vi "Update Configuration with Existing Modules.vi"(7 "Module IDs":string[](array[string]), 8 "error in":errorcluster, 9 "default error responses":T1={"unknown"={"clear"=TRUE, "notify"=TRUE, "log"=FALSE, "remove module"=FALSE, "abort engine"=FALSE, "go to safe state"=FALSE, "recover module"=FALSE}, "trivial"={"clear"=TRUE, "notify"=TRUE, "log"=FALSE, "remove module"=FALSE, "abort engine"=FALSE, "go to safe state"=FALSE, "recover module"=FALSE}, "critical"={"clear"=TRUE, "notify"=TRUE, "log"=FALSE, "remove module"=FALSE, "abort engine"=FALSE, "go to safe state"=FALSE, "recover module"=FALSE}, "recoverable"={"clear"=TRUE, "notify"=TRUE, "log"=FALSE, "remove module"=FALSE, "abort engine"=FALSE, "go to safe state"=FALSE, "recover module"=FALSE}}, 10 "Default Module Decimation":T3={"Decimation"=1, "Offset"=0, "sort order"=0, "async?"=FALSE}, 11 "Standard Engine Configuration in":refnum<class "Standard Engine Configuration.lvclass">) -> (0 "error out":errorcluster, 3 "Standard Engine Configuration out":refnum<class "Standard Engine Configuration.lvclass">)   [LabVIEW 2013, in "Standard Engine Configuration.lvclass"]
doc: "This VI synchronizes its module specific configuration information with the list of modules specified by 'Module IDs'. \n\nIf more modules are specified in 'Module IDs' than exist already in the module-specific configuration, than a new element is created for each new Module ID based on the 'Default Module Decimation' and 'Default Module Error Configuration' inputs. \n\nIf the module specific configuration contains elements not present in the 'Module IDs' input, the additional configurations are deleted."
uses:
  Standard Engine Configuration.lvclass
  Module Decimation.ctl
  Runtime/error responses.ctl
  error options.ctl
  Standard Engine Configuration.lvclass/Standard Engine Configuration.ctl
  Find Module Specific Config.vi
  <vilib>/NI/Configuration Framework/error generator/NISE_error generator.vi
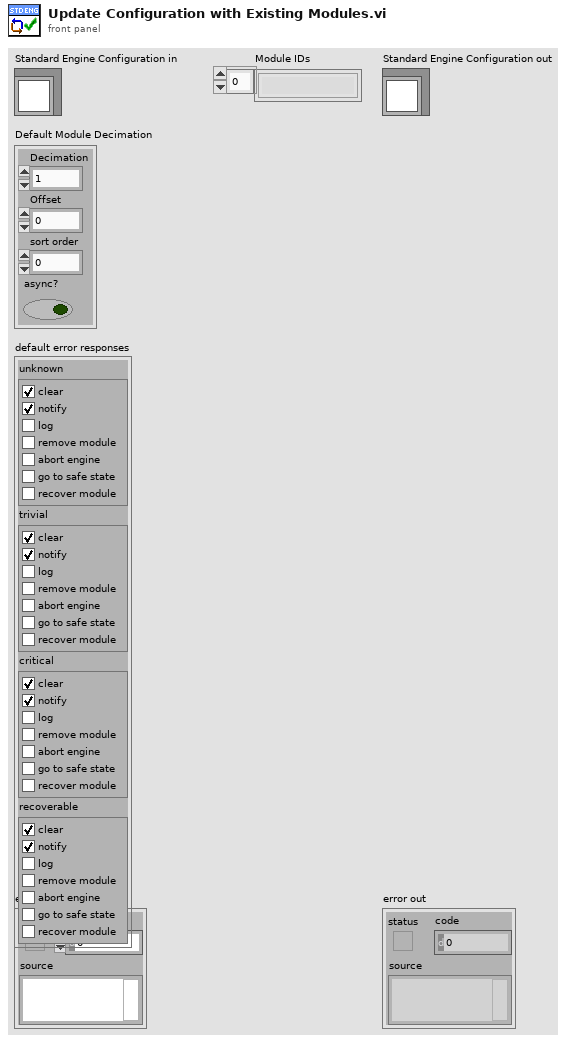
[diagram p1: front panel]
types:
  T1 = typedef "Standard Engine Configuration.lvclass/error responses.ctl" = cluster{"unknown":T2, "trivial":T2, "critical":T2, "recoverable":T2}
  T2 = typedef "Standard Engine Configuration.lvclass/error options.ctl" = cluster{"clear":bool, "notify":bool, "log":bool, "remove module":bool, "abort engine":bool, "go to safe state":bool, "recover module":bool}
  T3 = typedef "Standard Engine Configuration.lvclass/Module Decimation.ctl" = cluster{"Decimation":u16, "Offset":u16, "sort order":i32, "async?":bool}
  T4 = typedef "Standard Engine Configuration.lvclass/Module Specific Configuration.ctl" = cluster{"Module ID":string, "Module Decimation":T3, "error tag":string, "error responses":T1}
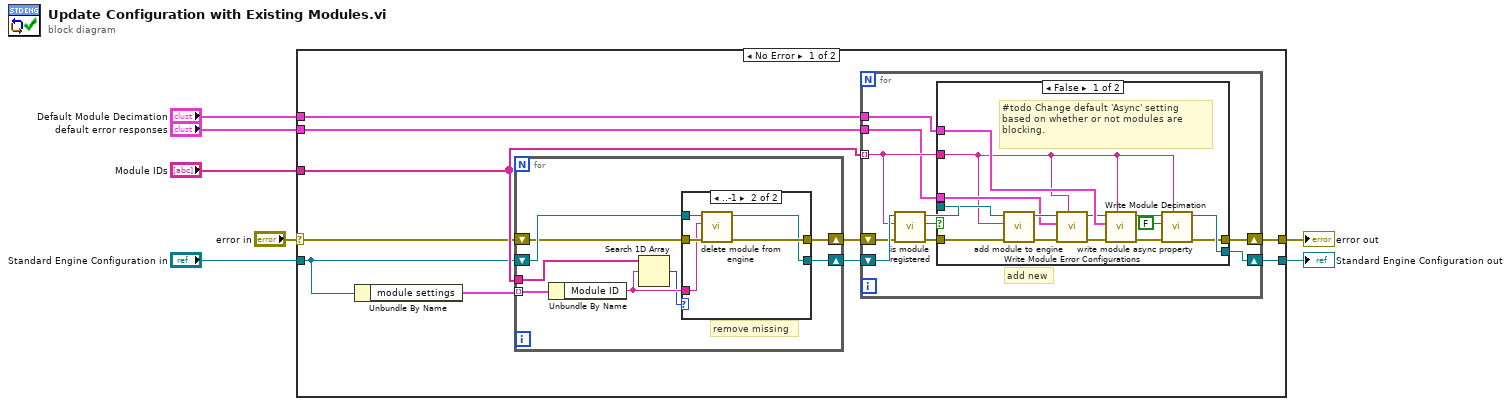
[diagram p0: block diagram]
diagram:
  n1 = case shown="No Error" "error in" {
    selector: "error in" -> [w11 w60]
    tunnel: [w15 w60] -> w6
    tunnel: [w16 w59] -> w4
    tunnel: "Standard Engine Configuration in" -> [w12 w59]
    tunnel: "Module IDs" -> [w13 _]
    tunnel: "Default Module Decimation" -> [w17 _]
    tunnel: "default error responses" -> [w8 _]
    frame No Error {
      n2 = Unbundle By Name(w12) -> ("module settings"=w14:T4[])
      n3 = for {
        tunnel: w14 -> [w25] mode=indexing
        tunnel: w13 -> [w24]
        shift-right: [w20] -> w10
        shift-left: w12 -> [w23]
        shift-right: [w21] -> w9
        shift-left: w11 -> [w22]
        # "remove missing"
        n4 = Unbundle By Name(w25) -> ("Module ID"=w19:string)
        n5 = Search 1D Array(1D array=w24, element=w19) -> (index of element=w18:i32)  [unwired: 1 in]
        n6 = case shown="..-1" w18 {
          tunnel: w23 -> [w27 w32]
          tunnel: w22 -> [w26 w31]
          tunnel: [w26 w30] -> w21
          tunnel: [w27 w29] -> w20
          tunnel: w19 -> [_ w28]
          frame 0.. {
          }
          frame ..-1 {
            n7 = call-dynamic "delete module from engine.vi"("error in"=w31, "module ID"=w28, "Standard Engine Configuration in"=w32) -> ("error out"=w30:errorcluster, "Standard Engine Configuration out"=w29:refnum<class "Standard Engine Configuration.lvclass">)  [unwired: 7 in]
          }
        }
      }
      n8 = for {
        shift-right: [w38] -> w15
        shift-left: w9 -> [w41]
        shift-right: [w39] -> w16
        shift-left: w10 -> [w42]
        tunnel: w13 -> [w36] mode=indexing
        tunnel: w17 -> [w34]
        tunnel: w8 -> [w33]
        # "add new"
        n9 = call-dynamic "is module registered.vi"("error in"=w41, "module ID"=w36, "engine configuration in"=w42) -> ("error out"=w37:errorcluster, "registered?"=w35:bool, "engine configuration out"=w40:refnum<class "Standard Engine Configuration.lvclass">)  [unwired: 6 in]
        n10 = case shown="False" w35 {
          tunnel: w40 -> [w56 w58]
          tunnel: [w45 w58] -> w39
          tunnel: [w44 w57] -> w38
          tunnel: w37 -> [w55 w57]
          tunnel: w36 -> [w46 _]
          tunnel: w34 -> [w52 _]
          tunnel: w33 -> [w49 _]
          frame False {
            # "#todo Change default 'Async' setting based on whether or not modules are blocking."
            n11 = call-dynamic "add module to engine.vi"("error in"=w55, "module ID"=w46, "Standard Engine Configuration in"=w56) -> ("error out"=w53:errorcluster, "Standard Engine Configuration out"=w54:refnum<class "Standard Engine Configuration.lvclass">)  [unwired: 7 in]
            n12 = call "Write Module Error Configurations.vi"("Module ID"=w46, "error in"=w53, "error responses"=w49, "Standard Engine Repo Data in"=w54) -> ("error out"=w51:errorcluster, "Standard Engine Repo Data out"=w50:refnum<class "Standard Engine Configuration.lvclass">)  [unwired: 6 in]
            n13 = call "Write Module Decimation.vi"("Module ID"=w46, "error in"=w51, "Module Decimation"=w52, "Standard Engine Repo Data in"=w50) -> ("error out"=w47:errorcluster, "Standard Engine Repo Data out"=w48:refnum<class "Standard Engine Configuration.lvclass">)  [unwired: 6 in]
            n14 = call "write module async property.vi"("Module ID"=w46, "error in"=w47, "async?"=FALSE, "Standard Engine Repo Data in"=w48) -> ("error out"=w44:errorcluster, "Standard Engine Repo Data out"=w45:refnum<class "Standard Engine Configuration.lvclass">)  [unwired: 6 in]
          }
          frame True {
          }
        }
      }
    }
    frame Error {
    }
  }
  "error out" <- w6
  "Standard Engine Configuration out" <- w4
